vi "20.Evd.7_Ask.4.vi"() -> ()   [LabVIEW 2025]
panel:
  in  "stop":bool
  in  "Birth Date":string[](array[string])=["1990", "1985", "1992", "1988", "1995"]
  in  "Last Name":string[](array[string])=["Smith", "Brown", "Johnson", "Davis", "Wilson"]
  in  "Name":string[](array[string])=["John", "Emily", "Michael", "Sarah", "David"]
  out "Result":string
  in  "Name":string
  in  "Element Category":string
  # "Taxpayer Information Finder"
  # "Select display of Registered user data\n\n-name\n-lastname\n-birthdate\n-all data"
  # "Numeric data table"
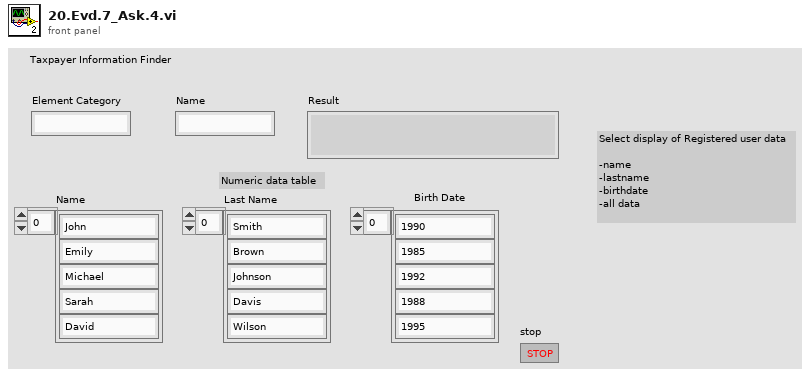
[diagram p1: front panel]
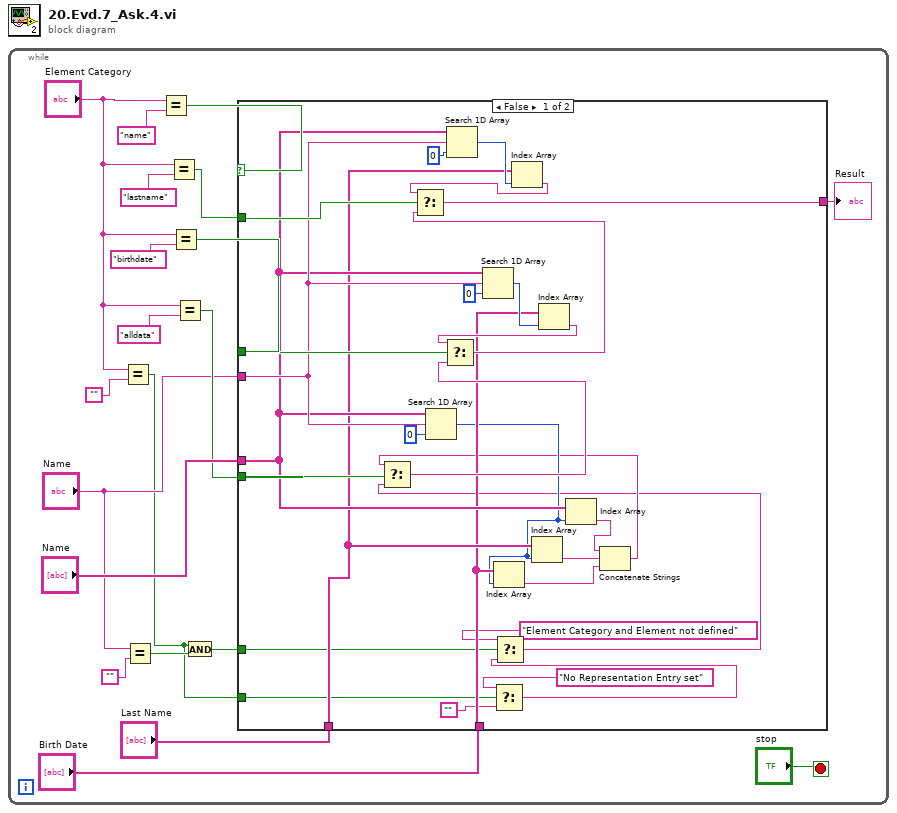
[diagram p0: block diagram]
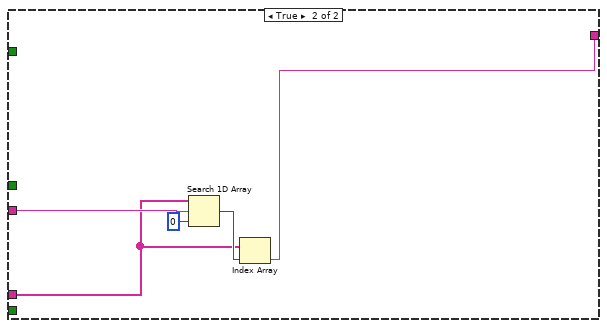
[diagram p2: hidden frame]
diagram:
  n1 = while {
    stop <- "stop" stop-if-true
    n2 = Equal?(x="Element Category", y="") -> (x = y?=w2:bool)
    n3 = Equal?(x="Name", y="") -> (x = y?=w4:bool)
    n4 = Equal?(x="Element Category", y="name") -> (x = y?=w16:bool)
    n5 = Equal?(x="Element Category", y="lastname") -> (x = y?=w13:bool)
    n6 = Equal?(x="Element Category", y="birthdate") -> (x = y?=w12:bool)
    n7 = Equal?(x="Element Category", y="alldata") -> (x = y?=w9:bool)
    n8 = And(x=w2, y=w4) -> (x .and. y?=w3:bool)
    n9 = case shown="False" w16 {
      tunnel: "Name" -> [w35 w51]
      tunnel: "Name" -> [w39 w52]
      tunnel: [w45 w50] -> w14
      tunnel: w13 -> [w49 _]
      tunnel: w12 -> [w44 _]
      tunnel: "Last Name" -> [w33 _]
      tunnel: "Birth Date" -> [w31 _]
      tunnel: w9 -> [w37 _]
      tunnel: w3 -> [w27 _]
      tunnel: w2 -> [w24 _]
      frame False {
        n10 = Search 1D Array(1D array=w35, element=w39, start index (0)=0) -> (index of element=w30:i32)
        n11 = Search 1D Array(1D array=w35, element=w39, start index (0)=0) -> (index of element=w48:i32)
        n12 = Search 1D Array(1D array=w35, element=w39, start index (0)=0) -> (index of element=w42:i32)
        n13 = Index Array(array=w31, index=w30) -> (element=w29:string)
        n14 = Select(t="No Representation Entry set", s=w24, f="") -> (s? t:f=w23:string)
        n15 = Select(t="Element Category and Element not defined", s=w27, f=w23) -> (s? t:f=w26:string)
        n16 = Index Array(array=w33, index=w48) -> (element=w46:string)
        n17 = Index Array(array=w33, index=w30) -> (element=w32:string)
        n18 = Index Array(array=w31, index=w42) -> (element=w41:string)
        n19 = Index Array(array=w35, index=w30) -> (element=w34:string)
        n20 = Concatenate Strings(w34, w32, w29) -> (w28:string)
        n21 = Select(t=w28, s=w37, f=w26) -> (s? t:f=w36:string)
        n22 = Select(t=w41, s=w44, f=w36) -> (s? t:f=w40:string)
        n23 = Select(t=w46, s=w49, f=w40) -> (s? t:f=w45:string)
      }
      frame True {
        n24 = Search 1D Array(1D array=w51, element=w52, start index (0)=0) -> (index of element=w54:i32)
        n25 = Index Array(array=w51, index=w54) -> (element=w50:string)
      }
    }
    "Result" <- w14
  }
